vi "Are Keys Down.vi"(7 "Require All Keys? (T)":bool=TRUE, 8 "error in":errorcluster, 10 "Keys":T1[](array[typedef]), 11 "Fallback Value (Mac only)":bool) -> (0 "error out":errorcluster, 3 "Are Keys Down?":bool)   [LabVIEW 2020, in "Execution UI.lvclass"]
doc: "Returns whether a list of keyboard <b>Keys</b> are down (currently being pressed).\n\nIf <b>Require All Keys?</b> is true (default), returns whether ALL of the <b>Keys</b> are down.\nIf <b>Require All Keys?</b> is false, returns whether ANY of the <b>Keys</b> are down.\n\nSince the functions used internally are not supported on Mac, there must be a <b>Fallback Value</b> obtained by a different method (e.g. through UI event data nodes).\n\nThis function has been added to address issue <b>#48</b> of missed key events when the VI loses the focus to e.g. a modal dialog."
uses:
  Execution UI.lvclass
  TypeDefs/Virtual Key.ctl
  <vilib>/Utility/inputDevices.llb/keyboardAcquire.vi
  <vilib>/Utility/inputDevices.llb/closeKeyboard.vi
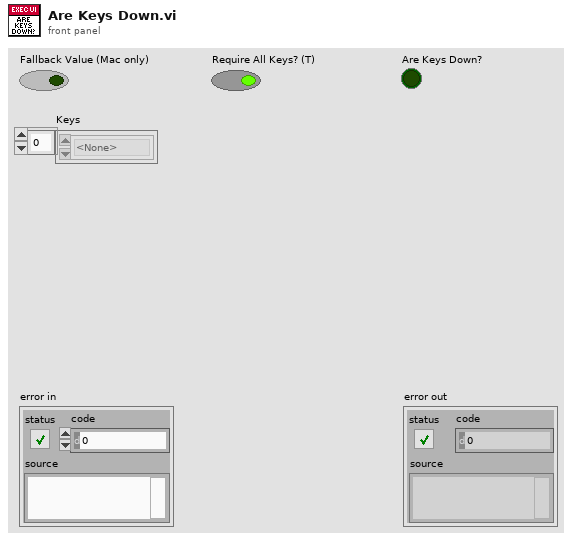
[diagram p1: front panel]
types:
  T1 = typedef "Execution UI.lvclass/Virtual Key.ctl" = enum16{"<None>", "Shift", "Ctrl", "Alt"}
  T2 = enum16{"0", "1", "2", "3", "4", "5", "6", "7", "8", "9", "A", "B", "C", "D", "E", "F", "G", "H", "I", "J", "K", "L", "M", "N", "O", "P", "Q", "R", "S", "T", "U", "V", "W", "X", "Y", "Z", "F1", "F2", "F3", "F4", "F5", "F6", "F7", "F8", "F9", "F10", "F11", "F12", "F13", "F14", "F15", "ADD", "BACK", "BACKSLASH", "CAPITAL", "COMMA", "DECIMAL", "DELETE", "DIVIDE", "DOWN", "END", "EQUALS", "ESCAPE", "GRAVE (`)", "HOME", "INSERT", "LBRACKET", "LCONTROL", "LEFT", "L ALT", "LSHIFT", "LWIN", "MINUS", "MULTIPLY", "NEXT", "NUMLOCK", "NUMPAD_0", "NUMPAD_1", "NUMPAD_2", "NUMPAD_3", "NUMPAD_4", "NUMPAD_5", "NUMPAD_6", "NUMPAD_7", "NUMPAD_8", "NUMPAD_9", "PAUSE", "PERIOD", "PRIOR (PG UP)", "RBRACKET", "RCONTROL", "RETURN", "RIGHT", "R ALT", "RSHIFT", "RWIN", "SCROLL", "SEMICOLON", "SLASH", "SPACE", "SUBTRACT", "TAB", "UP", "ENTER (num pad)", "' (quote)"}[]
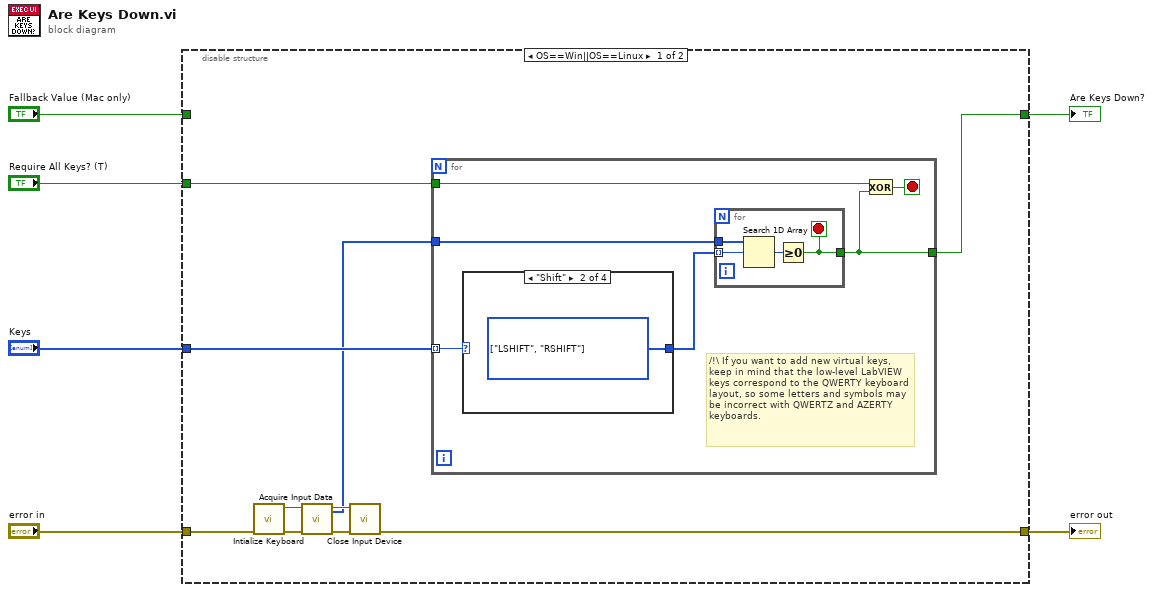
[diagram p0: block diagram]
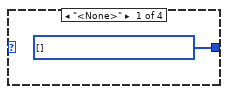
[diagram p2: hidden frame]
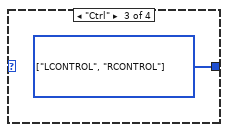
[diagram p3: hidden frame]
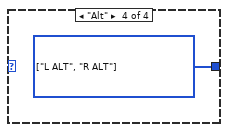
[diagram p4: hidden frame]
diagram:
  n1 = disable-structure shown="OS==Win||OS==Linux" {
    disable-tunnel: "error in" -> [w16 w32]
    disable-tunnel: [w12 w32] -> w5
    disable-tunnel: [w9 w31] -> w4
    disable-tunnel: "Fallback Value (Mac only)" -> [_ w31]
    disable-tunnel: "Keys" -> [w10 _]
    disable-tunnel: "Require All Keys? (T)" -> [w8 _]
    frame condition #0 (active) {
      n2 = call <vilib>:"Intialize Keyboard.vi"("error in (no error)"=w16) -> ("error out"=w15:errorcluster, "device ID"=w14:refnum<k1>)  [unwired: 9 in]
      n3 = call-poly <vilib>:"Acquire Input Data.vi"("device ID"=w14, "error in (no error)"=w15) -> ("device ID"=w11:refnum<k1>, "keys pressed"=w7:T2, "error out"=w13:errorcluster)  [unwired: 15 in]
      n4 = call-poly <vilib>:"Close Input Device.vi"("error in (no error)"=w13, "device ID"=w11) -> ("error out"=w12:errorcluster)  [unwired: 8 in]
      n5 = for {
        tunnel: w7 -> [w22]
        tunnel: w10 -> [w21] mode=indexing
        tunnel: [w18] -> w9
        tunnel: w8 -> [w19]
        stop <- w17 stop-if-true
        # "/!\\ If you want to add new virtual keys, keep in mind that the low-level LabVIEW keys correspond to the QWERTY keyboard layout, so some letters and symbols may be incorrect with QWERTZ and AZERTY keyboards."
        n6 = case shown="\"Shift\"" w21 {
          tunnel: [w23 w24 w25 w26] -> w20
          frame "<None>" {
            w23 = T2 [] items=["0", "1", "2", "3", "4", "5", "6", "7", "8", "9", "A", "B", "C", "D", "E", "F", "G", "H", "I", "J", "K", "L", "M", "N", "O", "P", "Q", "R", "S", "T", "U", "V", "W", "X", "Y", "Z", "F1", "F2", "F3", "F4", "F5", "F6", "F7", "F8", "F9", "F10", "F11", "F12", "F13", "F14", "F15", "ADD", "BACK", "BACKSLASH", "CAPITAL", "COMMA", "DECIMAL", "DELETE", "DIVIDE", "DOWN", "END", "EQUALS", "ESCAPE", "GRAVE (`)", "HOME", "INSERT", "LBRACKET", "LCONTROL", "LEFT", "L ALT", "LSHIFT", "LWIN", "MINUS", "MULTIPLY", "NEXT", "NUMLOCK", "NUMPAD_0", "NUMPAD_1", "NUMPAD_2", "NUMPAD_3", "NUMPAD_4", "NUMPAD_5", "NUMPAD_6", "NUMPAD_7", "NUMPAD_8", "NUMPAD_9", "PAUSE", "PERIOD", "PRIOR (PG UP)", "RBRACKET", "RCONTROL", "RETURN", "RIGHT", "R ALT", "RSHIFT", "RWIN", "SCROLL", "SEMICOLON", "SLASH", "SPACE", "SUBTRACT", "TAB", "UP", "ENTER (num pad)", "' (quote)"]
          }
          frame "Shift" {
            w24 = T2 [enum."LSHIFT", enum."RSHIFT"] items=["0", "1", "2", "3", "4", "5", "6", "7", "8", "9", "A", "B", "C", "D", "E", "F", "G", "H", "I", "J", "K", "L", "M", "N", "O", "P", "Q", "R", "S", "T", "U", "V", "W", "X", "Y", "Z", "F1", "F2", "F3", "F4", "F5", "F6", "F7", "F8", "F9", "F10", "F11", "F12", "F13", "F14", "F15", "ADD", "BACK", "BACKSLASH", "CAPITAL", "COMMA", "DECIMAL", "DELETE", "DIVIDE", "DOWN", "END", "EQUALS", "ESCAPE", "GRAVE (`)", "HOME", "INSERT", "LBRACKET", "LCONTROL", "LEFT", "L ALT", "LSHIFT", "LWIN", "MINUS", "MULTIPLY", "NEXT", "NUMLOCK", "NUMPAD_0", "NUMPAD_1", "NUMPAD_2", "NUMPAD_3", "NUMPAD_4", "NUMPAD_5", "NUMPAD_6", "NUMPAD_7", "NUMPAD_8", "NUMPAD_9", "PAUSE", "PERIOD", "PRIOR (PG UP)", "RBRACKET", "RCONTROL", "RETURN", "RIGHT", "R ALT", "RSHIFT", "RWIN", "SCROLL", "SEMICOLON", "SLASH", "SPACE", "SUBTRACT", "TAB", "UP", "ENTER (num pad)", "' (quote)"]
          }
          frame "Ctrl" {
            w25 = T2 [enum."LCONTROL", enum."RCONTROL"] items=["0", "1", "2", "3", "4", "5", "6", "7", "8", "9", "A", "B", "C", "D", "E", "F", "G", "H", "I", "J", "K", "L", "M", "N", "O", "P", "Q", "R", "S", "T", "U", "V", "W", "X", "Y", "Z", "F1", "F2", "F3", "F4", "F5", "F6", "F7", "F8", "F9", "F10", "F11", "F12", "F13", "F14", "F15", "ADD", "BACK", "BACKSLASH", "CAPITAL", "COMMA", "DECIMAL", "DELETE", "DIVIDE", "DOWN", "END", "EQUALS", "ESCAPE", "GRAVE (`)", "HOME", "INSERT", "LBRACKET", "LCONTROL", "LEFT", "L ALT", "LSHIFT", "LWIN", "MINUS", "MULTIPLY", "NEXT", "NUMLOCK", "NUMPAD_0", "NUMPAD_1", "NUMPAD_2", "NUMPAD_3", "NUMPAD_4", "NUMPAD_5", "NUMPAD_6", "NUMPAD_7", "NUMPAD_8", "NUMPAD_9", "PAUSE", "PERIOD", "PRIOR (PG UP)", "RBRACKET", "RCONTROL", "RETURN", "RIGHT", "R ALT", "RSHIFT", "RWIN", "SCROLL", "SEMICOLON", "SLASH", "SPACE", "SUBTRACT", "TAB", "UP", "ENTER (num pad)", "' (quote)"]
          }
          frame "Alt" {
            w26 = T2 [enum."L ALT", enum."R ALT"] items=["0", "1", "2", "3", "4", "5", "6", "7", "8", "9", "A", "B", "C", "D", "E", "F", "G", "H", "I", "J", "K", "L", "M", "N", "O", "P", "Q", "R", "S", "T", "U", "V", "W", "X", "Y", "Z", "F1", "F2", "F3", "F4", "F5", "F6", "F7", "F8", "F9", "F10", "F11", "F12", "F13", "F14", "F15", "ADD", "BACK", "BACKSLASH", "CAPITAL", "COMMA", "DECIMAL", "DELETE", "DIVIDE", "DOWN", "END", "EQUALS", "ESCAPE", "GRAVE (`)", "HOME", "INSERT", "LBRACKET", "LCONTROL", "LEFT", "L ALT", "LSHIFT", "LWIN", "MINUS", "MULTIPLY", "NEXT", "NUMLOCK", "NUMPAD_0", "NUMPAD_1", "NUMPAD_2", "NUMPAD_3", "NUMPAD_4", "NUMPAD_5", "NUMPAD_6", "NUMPAD_7", "NUMPAD_8", "NUMPAD_9", "PAUSE", "PERIOD", "PRIOR (PG UP)", "RBRACKET", "RCONTROL", "RETURN", "RIGHT", "R ALT", "RSHIFT", "RWIN", "SCROLL", "SEMICOLON", "SLASH", "SPACE", "SUBTRACT", "TAB", "UP", "ENTER (num pad)", "' (quote)"]
          }
        }
        n7 = for {
          tunnel: w22 -> [w30]
          tunnel: w20 -> [w29] mode=indexing
          tunnel: [w27] -> w18
          stop <- w27 stop-if-true
          n8 = Search 1D Array(1D array=w30, element=w29) -> (index of element=w28:i32)  [unwired: 1 in]
          n9 = Greater Or Equal To 0?(x=w28) -> (x >= 0?=w27:bool)
        }
        n10 = Exclusive Or(1:w18, 2:w19) -> (0:w17:bool)
      }
    }
    frame condition #1 {
      # "macOS implementation needed (then the fallback value can be removed)"
    }
  }
  "error out" <- w5
  "Are Keys Down?" <- w4
